vi "Start Triggers Time.vi"(0 "time.resources":T10, 5 "rx.parameters":T7={"rx.trigger select"=enum."Software", "rx.trigger enable"=FALSE, "rx.trigger sync enable"=FALSE, "rx 0.stream enable"=FALSE, "rx 1.stream enable"=FALSE, "rx.software trigger"=FALSE, "rx.reset"=FALSE, "rx.abort"=FALSE, "rx.samples to acquire"=0, "ddc parameters"=[{"output sample rate"=0.0, "delay"=0.0, "frequency shift"=0.0, "impairments"={"inline gain I"=0.0, "inline gain Q"=0.0, "cross gain I"=0.0, "cross gain Q"=0.0, "pre-gain offset I"=0.0, "pre-gain offset Q"=0.0, "post-gain offset I"=0.0, "post-gain offset Q"=0.0}, "phase"=0.0}, {"output sample rate"=0.0, "delay"=0.0, "frequency shift"=0.0, "impairments"={"inline gain I"=0.0, "inline gain Q"=0.0, "cross gain I"=0.0, "cross gain Q"=0.0, "pre-gain offset I"=0.0, "pre-gain offset Q"=0.0, "post-gain offset I"=0.0, "post-gain offset Q"=0.0}, "phase"=0.0}]} {"ddc parameters"."frequency shift" format="%#.48g"}, 7 "tx.parameters":T5={"tx.trigger select"=enum."Software", "tx.trigger enable"=FALSE, "tx.trigger sync enable"=FALSE, "tx 0.stream enable"=FALSE, "tx 1.stream enable"=FALSE, "tx.software trigger"=FALSE, "tx.reset"=FALSE, "tx.abort"=FALSE, "tx.samples to generate"=0, "duc parameters"=[{"frequency shift"=0.0, "impairments"={"inline gain I"=0.0, "inline gain Q"=0.0, "cross gain I"=0.0, "cross gain Q"=0.0, "pre-gain offset I"=0.0, "pre-gain offset Q"=0.0, "post-gain offset I"=0.0, "post-gain offset Q"=0.0}, "phase"=0.0, "input sample rate"=0.0, "gain"={"gain I"=0.0, "gain Q"=0.0}, "delay"=0.0}, {"frequency shift"=0.0, "impairments"={"inline gain I"=0.0, "inline gain Q"=0.0, "cross gain I"=0.0, "cross gain Q"=0.0, "pre-gain offset I"=0.0, "pre-gain offset Q"=0.0, "post-gain offset I"=0.0, "post-gain offset Q"=0.0}, "phase"=0.0, "input sample rate"=0.0, "gain"={"gain I"=0.0, "gain Q"=0.0}, "delay"=0.0}]} {"duc parameters"."frequency shift" format="%#.48g"}) -> (4 "rx.start trigger":bool, 6 "tx.start trigger":bool)   [LabVIEW 2015]
doc: "Generates start triggers for Rx and Tx. Start triggers are generated based on which trigger type is selected, whether the stream is enabled, whether triggers are enabled, and whether the triggers are to be synchronized across multiple devices.\n\n<B>Input Parameters</B>\n\n<B>enable stream</B> controls the output of a 'start trigger'.\n\n<B>enable trigger</B> controls the output of a 'start trigger'.\n\n<B>enable trigger sync</B> to synchronize a 'start trigger' between multiple devices. The master device sends the 'start trigger' to all the slave devices. If enabled, the slave devices ignore the 'trigger select' because the 'start trigger' from the master device is used instead.\n\n<B>trigger select</B> picks which source to use as the 'start trigger'.\n\n<B>Output Parameters</B>\n\n<B>rx.start trigger</B> is the signal to use at the 'start trigger' for the Rx data path.\n\n<B>tx.start trigger</B> is the signal to use at the 'start trigger' for the Tx data path."
uses:
  <instrlib>/niUsrpRio/Time/v1/FPGA/Private/Time Resources.ctl
  <instrlib>/niUsrpRio/Time/v1/FPGA/Private/Future Event Resources.ctl
  Host/SubVIs/Start Trigger.ctl
  DDC Parameters.ctl
  <instrlib>/_niInstr/DSP/v1/Shared/Public/IQ Impairments.ctl
  DUC Parameters.ctl
  <instrlib>/_niInstr/DSP/v1/Shared/Public/IQ Gain.ctl
  <instrlib>/niUsrpRio/Time/v1/FPGA/niUsrpRio Time v1 FPGA.lvlib
  <instrlib>/_niInstr/DSP/v1/Shared/niInstr DSP v1 Shared.lvlib
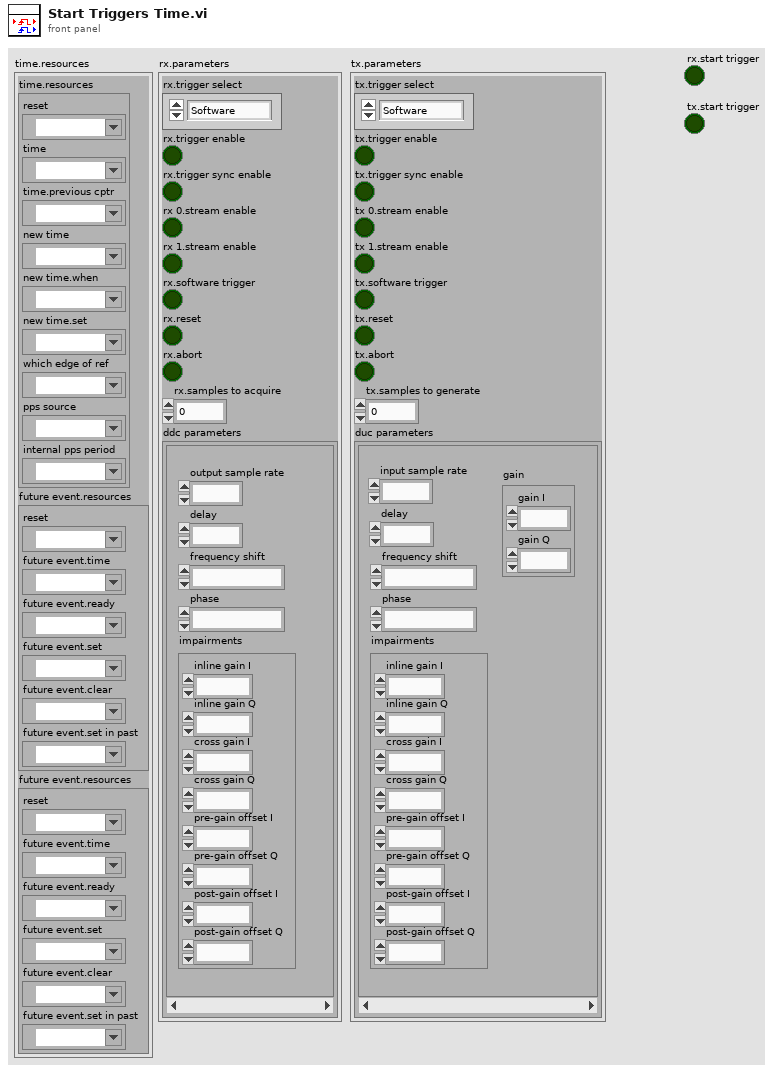
[diagram p1: front panel]
types:
  T1 = typedef "Start Trigger.ctl" = enum8{"Software", "Digital Edge", "Rx Start Trigger", "Tx Start Trigger", "Immediate", "Future Time Event"}
  T2 = typedef "DUC Parameters.ctl" = cluster{"frequency shift":fxp<+/-,48,0>, "impairments":T3, "phase":fxp<+/-,21,0>, "input sample rate":fxp<+,48,1>, "gain":T4, "delay":fxp<+/-,18,0>}
  T3 = typedef "niInstr DSP v1 Shared.lvlib/IQ Impairments.ctl" = cluster{"inline gain I":fxp<+/-,18,1>, "inline gain Q":fxp<+/-,18,1>, "cross gain I":fxp<+/-,18,1>, "cross gain Q":fxp<+/-,18,1>, "pre-gain offset I":fxp<+/-,18,1>, "pre-gain offset Q":fxp<+/-,18,1>, "post-gain offset I":fxp<+/-,18,1>, "post-gain offset Q":fxp<+/-,18,1>}
  T4 = typedef "niInstr DSP v1 Shared.lvlib/IQ Gain.ctl" = cluster{"gain I":fxp<+/-,24,3>, "gain Q":fxp<+/-,24,3>}
  T5 = cluster{"tx.trigger select":T1, "tx.trigger enable":bool, "tx.trigger sync enable":bool, "tx 0.stream enable":bool, "tx 1.stream enable":bool, "tx.software trigger":bool, "tx.reset":bool, "tx.abort":bool, "tx.samples to generate":u32, "duc parameters":T2[]}
  T6 = typedef "DDC Parameters.ctl" = cluster{"output sample rate":fxp<+,48,1>, "delay":fxp<+/-,16,0>, "frequency shift":fxp<+/-,48,0>, "impairments":T3, "phase":fxp<+/-,21,0>}
  T7 = cluster{"rx.trigger select":T1, "rx.trigger enable":bool, "rx.trigger sync enable":bool, "rx 0.stream enable":bool, "rx 1.stream enable":bool, "rx.software trigger":bool, "rx.reset":bool, "rx.abort":bool, "rx.samples to acquire":u32, "ddc parameters":T6[]}
  T8 = typedef "niUsrpRio Time v1 FPGA.lvlib/Time Resources.ctl" = cluster{"reset":refnum<k21>, "time":refnum<k21>, "time.previous cptr":refnum<k21>, "new time":refnum<k21>, "new time.when":refnum<k21>, "new time.set":refnum<k21>, "which edge of ref":refnum<k21>, "pps source":refnum<k21>, "internal pps period":refnum<k21>}
  T9 = typedef "niUsrpRio Time v1 FPGA.lvlib/Future Event Resources.ctl" = cluster{"reset":refnum<k21>, "future event.time":refnum<k21>, "future event.ready":refnum<k21>, "future event.set":refnum<k21>, "future event.clear":refnum<k21>, "future event.set in past":refnum<k21>}
  T10 = cluster{"time.resources":T8, "future event.resources":T9, "future event.resources":T9}
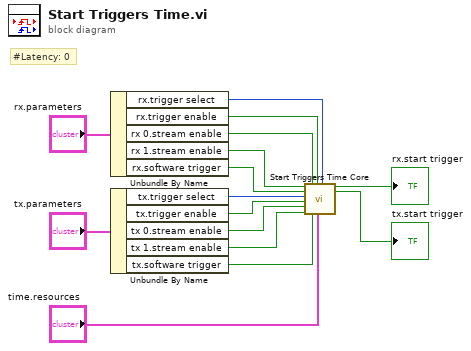
[diagram p0: block diagram]
diagram:
  # "#Latency: 0"
  n1 = Unbundle By Name("rx.parameters") -> ("rx.trigger select"=w11:T1, "rx.trigger enable"=w10:bool, "rx 0.stream enable"=w9:bool, "rx 1.stream enable"=w8:bool, "rx.software trigger"=w7:bool)
  n2 = Unbundle By Name("tx.parameters") -> ("tx.trigger select"=w5:T1, "tx.trigger enable"=w4:bool, "tx 0.stream enable"=w3:bool, "tx 1.stream enable"=w2:bool, "tx.software trigger"=w1:bool)
  n3 = call "Start Triggers Time Core.vi"("rx 1.stream enable"=w8, "rx.software trigger"=w7, "tx.trigger select"=w5, "tx.trigger enable"=w4, "tx 0.stream enable"=w3, "tx 1.stream enable"=w2, "rx 0.stream enable"=w9, "tx.software trigger"=w1, "rx.trigger enable"=w10, "time.resources"="time.resources", "rx.trigger select"=w11) -> ("rx.start trigger"=→"rx.start trigger":bool, "tx.start trigger"=→"tx.start trigger":bool)  [unwired: 7 in]
